vi "FRIC_navX_Get_Registry.vi"(7 "Update":bool, 9 "Connected?":bool, 11 "Registry (in)":u8[](array[numeric])) -> (1 "Connected?":bool, 3 "Registry (out)":u8[](array[numeric]))   [LabVIEW 2015, in "navX AE v1.lvlib"]
uses:
  navX AE v1.lvlib
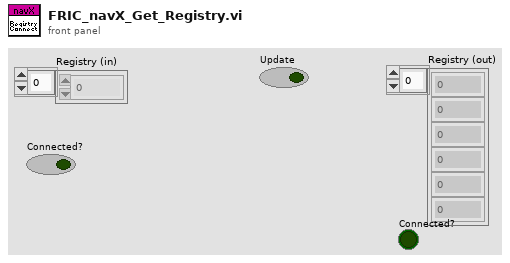
[diagram p1: front panel]
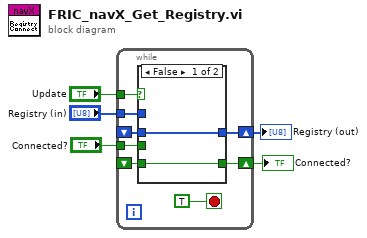
[diagram p0: block diagram]
diagram:
  n1 = while {
    shift-right: [w10] -> w3
    shift-left: _ -> [w9]
    tunnel: "Update" -> [w12]
    tunnel: "Registry (in)" -> [w11]
    shift-right: [w7] -> w1
    shift-left: _ -> [w6]
    tunnel: "Connected?" -> [w8]
    stop <- TRUE stop-if-true
    n2 = case shown="False" w12 {
      tunnel: w11 -> [_ w17]
      tunnel: [w15 w17] -> w10
      tunnel: w9 -> [w15 _]
      tunnel: w8 -> [_ w16]
      tunnel: [w14 w16] -> w7
      tunnel: w6 -> [w14 _]
      frame False {
      }
      frame True {
      }
    }
  }
  "Registry (out)" <- w3
  "Connected?" <- w1
